vi "ABB #s to strings.vi"(7 "# type":enum16{"Float", "Relative time HH:MM"}(ring), 9 "precisions":i32[](array[numeric]), 10 "Precision":i32, 11 "Numbers in":dbl[](array[numeric])) -> (3 "Strings out":string[](array[string]))   [LabVIEW 2017]
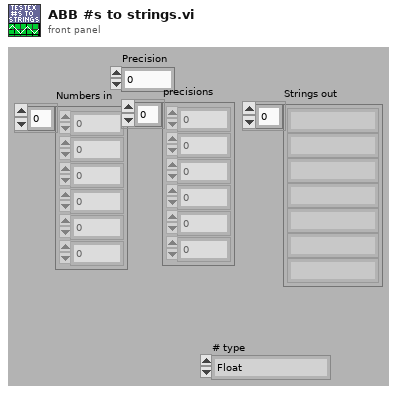
[diagram p1: front panel]
types:
  T1 = cluster{"Integer":i32, "Dbl":dbl, "String":string, "Boolean":bool}
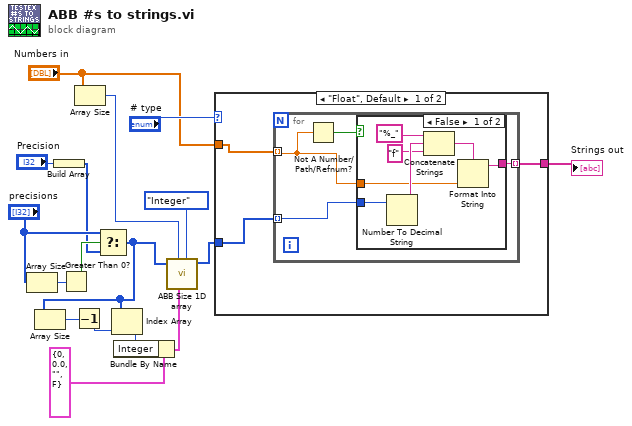
[diagram p0: block diagram]
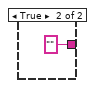
[diagram p2: hidden frame]
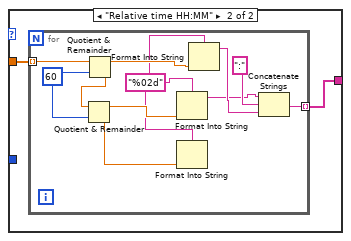
[diagram p3: hidden frame]
diagram:
  n1 = Array Size(array="precisions") -> (size(s)=w15:i32)
  n2 = Build Array("Precision") -> (w11:i32[])
  n3 = Greater Than 0?(x=w15) -> (x > 0?=w14:bool)
  n4 = Array Size(array="Numbers in") -> (size(s)=w7:i32)
  n5 = Select(t="precisions", s=w14, f=w11) -> (s? t:f=w3:i32[])
  n6 = Array Size(array=w3) -> (size(s)=w4:i32)
  n7 = Decrement(x=w4) -> (x-1=w2:i32)
  n8 = Index Array(array=w3, index=w2) -> (element=w1:i32)
  n9 = Bundle By Name(cluster=T1 {"Integer"=0, "Dbl"=0.0, "String"="", "Boolean"=FALSE} ("Default"), "Integer"=w1) -> (w6:T1)
  n10 = call "ABB Size 1D array.vi"("Type"=enum16{"Integer", "DBL", "STRING", "BOOLEAN"}."Integer", "Default"=w6, "Size"=w7, "Integer Array In"=w3) -> ("Integer Array Out"=w9:i32[])  [unwired: 4 in, 3 out]
  n11 = case shown="\"Float\", Default" "# type" {
    tunnel: "Numbers in" -> [w20 w34]
    tunnel: [w19 w33] -> w17
    tunnel: w9 -> [w18 _]
    frame "Float", Default {
      n12 = for {
        tunnel: w20 -> [w23] mode=indexing
        tunnel: [w24] -> w19 mode=indexing
        tunnel: w18 -> [w21] mode=indexing
        n13 = Not A Number/Path/Refnum?(number/path/refnum=w23) -> (NaN/Path/Refnum?=w22:bool)
        n14 = case shown="False" w22 {
          tunnel: [w31 ""] -> w24
          tunnel: w21 -> [w29 _]
          tunnel: w23 -> [w25 _]
          frame False {
            n15 = Number To Decimal String(number=w29) -> (decimal integer string=w28:string)  [unwired: 1 in]
            n16 = Concatenate Strings("%_" ("format string"), w28, "f" ("format string")) -> (w26:string)
            n17 = Format Into String(format string=w26, w25) -> (resulting string=w31:string)  [unwired: 2 in, 1 out]
          }
          frame True {
          }
        }
      }
    }
    frame "Relative time HH:MM" {
      n18 = for {
        tunnel: w34 -> [w45] mode=indexing
        tunnel: [w38] -> w33 mode=indexing
        w37 = "%02d" ("format string")
        w42 = 60 ("Number in")
        n19 = Quotient & Remainder(x=w45, y=w42) -> (x-y*floor(x/y)=w44:dbl, floor(x/y)=w43:dbl)
        n20 = Quotient & Remainder(x=w43, y=w42) -> (x-y*floor(x/y)=w41:dbl, floor(x/y)=w40:dbl)
        n21 = Format Into String(format string=w37, w41) -> (resulting string=w35:string)  [unwired: 2 in, 1 out]
        n22 = Format Into String(format string=w37, w40) -> ()  [unwired: 2 in, 2 out]
        n23 = Format Into String(format string=w37, w44) -> (resulting string=w36:string)  [unwired: 2 in, 1 out]
        n24 = Concatenate Strings(w35, ":", w36) -> (w38:string)
      }
    }
  }
  "Strings out" <- w17
